vi "Visit Nodes.vi"(7 "Order":T2, 8 "error in (no error)":errorcluster, 9 "User Data In":variant, 11 "AST in":refnum<class "AST.lvclass">) -> (0 "error out":errorcluster, 1 "User Data":variant, 3 "AST out":refnum<class "AST.lvclass">)   [LabVIEW 2020, in "PicoG-ParserLexer.lvlib" / "AST.lvclass"]
uses:
  AST.lvclass
  Outside Traversal Order.ctl
  PicoG-ParserLexer.lvlib
  Visitor VI.ctl
  Node/Node.lvclass
panel:
  in  "Visitor VI":T1
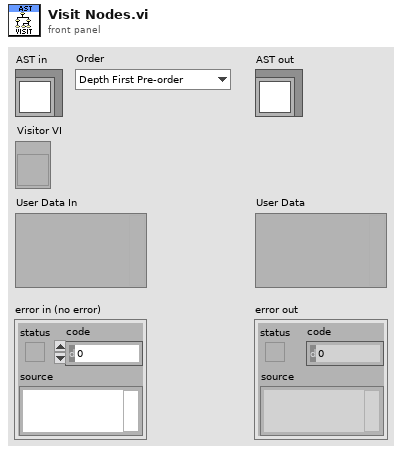
[diagram p1: front panel]
types:
  T1 = typedef "PicoG-ParserLexer.lvlib/AST.lvclass/Visitor VI.ctl" = refnum<vi>
  T2 = typedef "PicoG-ParserLexer.lvlib/Outside Traversal Order.ctl" = enum16{"Depth First Pre-order", "Depth First Post-order", "Breadth First Order"}
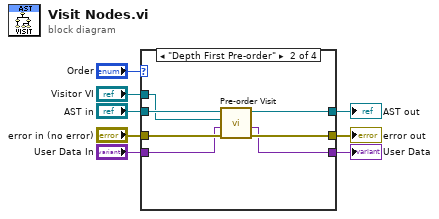
[diagram p0: block diagram]
diagram:
  n1 = case shown="\"Depth First Pre-order\"" "Order" {
    tunnel: "AST in" -> [w11 w18 _ _]
    tunnel: "error in (no error)" -> [w10 w16 _ _]
    tunnel: "User Data In" -> [w9 w13 _ _]
    tunnel: [w11 w17 _ _] -> w4
    tunnel: [w10 w15 _ _] -> w3
    tunnel: [w9 w12 _ _] -> w2
    tunnel: "Visitor VI" -> [_ w14 _ _]
    frame Default {
    }
    frame "Depth First Pre-order" {
      n2 = call "Pre-order Visit.vi"("error in (no error)"=w16, "User Data In"=w13, "Visitor VI"=w14, "AST in"=w18) -> ("error out"=w15:errorcluster, "User Data"=w12:variant, "AST out"=w17:refnum<class "AST.lvclass">)  [unwired: 5 in]
    }
    frame "Depth First Post-order" {
    }
    frame "Breadth First Order" {
    }
  }
  "error out" <- w3
  "AST out" <- w4
  "User Data" <- w2
